vi "GenAppMain.vi"() -> ()   [LabVIEW 2018]
doc: "DESCRIPTION\nGeneral Application \n\nVERSION\nD1:00\nFirst Release To customer\nDD/MM/YYYY\n\nTemplate D2:01\nMade lighter and simpler\n14-04-2020"
uses:
  SubVIs/Controls/SetupModeState.ctl
  <vilib>/event_ctls.llb/eventsource.ctl
  SubVIs/Controls/DisplayQCommand.ctl
  SubVIs/Controls/QueueCommand.ctl
  SubVIs/Controls/DisplayMessage.ctl
  SubVIs/Controls/Transition.ctl
  SubVIs/utilities/Error/ErrorCommand.ctl
  SubVIs/Controls/Tab.ctl
  SubVIs/Controls/StateMessage.ctl
  SubVIs/Error/ErrorMessage.ctl
  SubVIs/utilities/Config/System Config Data Manager Parameter.ctl
  SubVIs/utilities/Config/ConfigCommand.ctl
panel:
  in  "Stop":bool
  in  "Source":T1 items=["LabVIEW UI"=0, "ActiveX"=1, "User Event"=25]
  out "ErrorHandlingLoop":i32
  out "StateMachineLoop":i32
  out "Version":string
  out "Time":string
  out "UILoop":i32
  out "EventLoop":i32
  in  "Main Screen Tabs":enum32{"Main Screen"}(tab)
  out "Tab Control":T2(tab)
  in  "Error Loop":enum16{"Event Loop", "UI Q Loop", "State Loop"}(ring)
  in  "Generate Error":bool
  out "EngMode?":bool
  in  "Enter Password":string
  out "ConfigdB path":path
  in  "Home Button":bool
  in  "ErrorLog":bool
  in  "Clear Alarm":bool
  in  "ErrorLog":i32(listbox)
  out "Error":string
  out "ErrorIndicator":bool
  out "State":T3=enum."Initialising"
  in  "ViewError":bool
  out "Status":string
  in  "Start":bool
  in  "exit":bool
  # "GenAppMain"
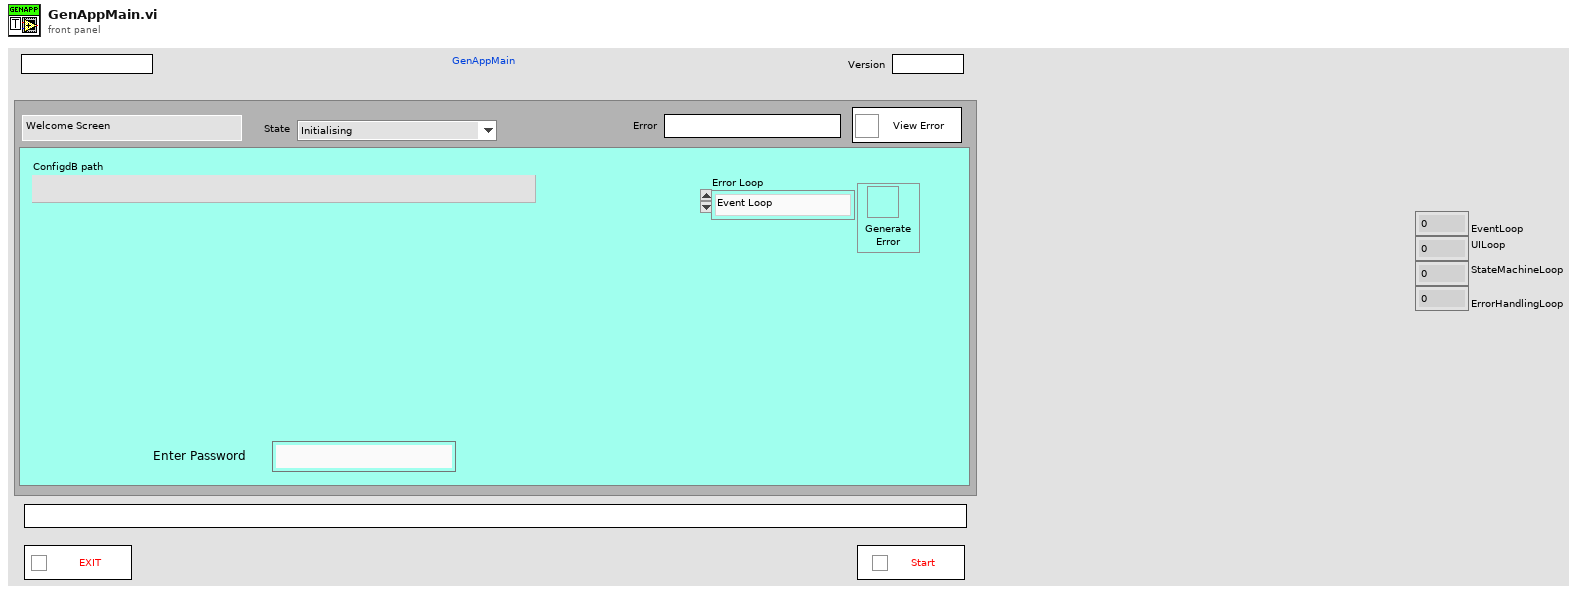
[diagram p1: front panel]
types:
  T1 = typedef "eventsource.ctl" = u32
  T2 = enum32{"Welcome Screen", "Eng Set Up", "Oppo Run Screen", "Eng Run Screen", "Test Report Screen", "Error"}
  T3 = typedef "SetupModeState.ctl" = enum16{"No State - Error", "Initialising", "Idling", "Running", "Erroring", "Exiting"}
  T4 = typedef "DisplayQCommand.ctl" = enum16{"No Command - Error", "Initialise", "Get Q Reference", "Add Item to Bottom", "Add Item to Top", "Flush Q", "Dequeue", "Peek Next Element", "Close"}
  T5 = typedef "QueueCommand.ctl" = enum16{"No Command - Error", "Initialise", "Add to Bottom", "Add To Top", "Get Ref", "Close"}
  T6 = typedef "ErrorCommand.ctl" = enum16{"No Command - Error", "Set to Dev Mode", "Set To Released Mode", "Set Error", "Log Error", "Throw Error", "Log & Throw Error", "Set Error Timed"}
  T7 = enum32{"invalid app kind", "Development System", "Run Time System", "Student Edition", "Embedded LabVIEW", "Evaluation", "Custom"}
  T8 = typedef "DisplayMessage.ctl" = enum16{"No Message - Ignore", "Display Message", "Set Tab", "Set Status", "Add Error Message", "Clear Error History", "Generate Error", "Set Idling Display", "Set Running Display", "Stop"}
  T9 = typedef "ErrorMessage.ctl" = enum16{"No Message - Ignore", "Display Message", "Stop"}
  T10 = typedef "StateMessage.ctl" = cluster{"Transition":T11, "variant":variant}
  T11 = typedef "Transition.ctl" = enum16{"No Transition - Error", "Initialise", "Login", "Authenticate", "Log on Fail", "Login Success", "Logout", "Generate Error", "Start", "Stop", "Exit"}
  T12 = typedef "ConfigCommand.ctl" = enum16{"No Command - Error", "Initialise Config SQLite", "Save Config", "Get Key", "Set Key", "Update Key", "Get Latest Config Data", "Get Config Data for Version", "Get Default Config Data"}
  T13 = typedef "System Config Data Manager Parameter.ctl" = enum16{"Eng Password", "DSN Connection", "User Password", "RunStatus", "InitialDataPath", "helpFilePath", "ErrorFilepath", "DatalogPath", "Hello"}
  T14 = typedef "Tab.ctl" = enum32{"Welcome Screen", "Eng Set Up", "Oppo Run Screen", "Eng Run Screen", "Test Report Screen", "Error"}
  T15 = typedef "lveventtype.ctl" = enum32{"Null", "Timeout", "Annotation Menu Selection", "Annotation Menu Selection?", "App Instance Close", "App Instance Close?", "Autoscale Range Change", "Bookmark Info Change", "Cell Edit", "Cell Edit?", "Cursor Grab", "Cursor Grab?", "Cursor Menu Selection", "Cursor Menu Selection?", "Cursor Move", "Cursor Release", "Data Change", "Direction Change", "Display State Change", "Drag Ended", "Drag Enter", "Drag Leave", "Drag Over", "Drag Source Update", "Drag Starting", "Drag Starting?", "Drop", "Exec State Change", "Key Down", "Key Down?", "Key Repeat", "Key Repeat?", "Key Up", "Listbox Double Click", "Menu Activation?", "Menu Selection (App)", "Menu Selection? (App)", "Menu Selection (User)", "Mouse Down", "Mouse Down?", "Mouse Enter", "Mouse Leave", "Mouse Move", "Mouse Up", "Mouse Wheel", "NI Security User Change (App)", "Pane Size", "Panel Close", "Panel Close?", "Panel Resize", "Plot Attribute Change", "Scale Range Change", "Shortcut Menu Activation?", "Shortcut Menu Selection (App)", "Shortcut Menu Selection? (App)", "Shortcut Menu Selection (User)", "Tree Double Click", "Tree Drag", "Tree Drag?", "Tree Drop", "Tree Drop?", "Tree Item Close", "Tree Item Close?", "Tree Item Open", "Tree Item Open?", "User Event", "Value Change"}
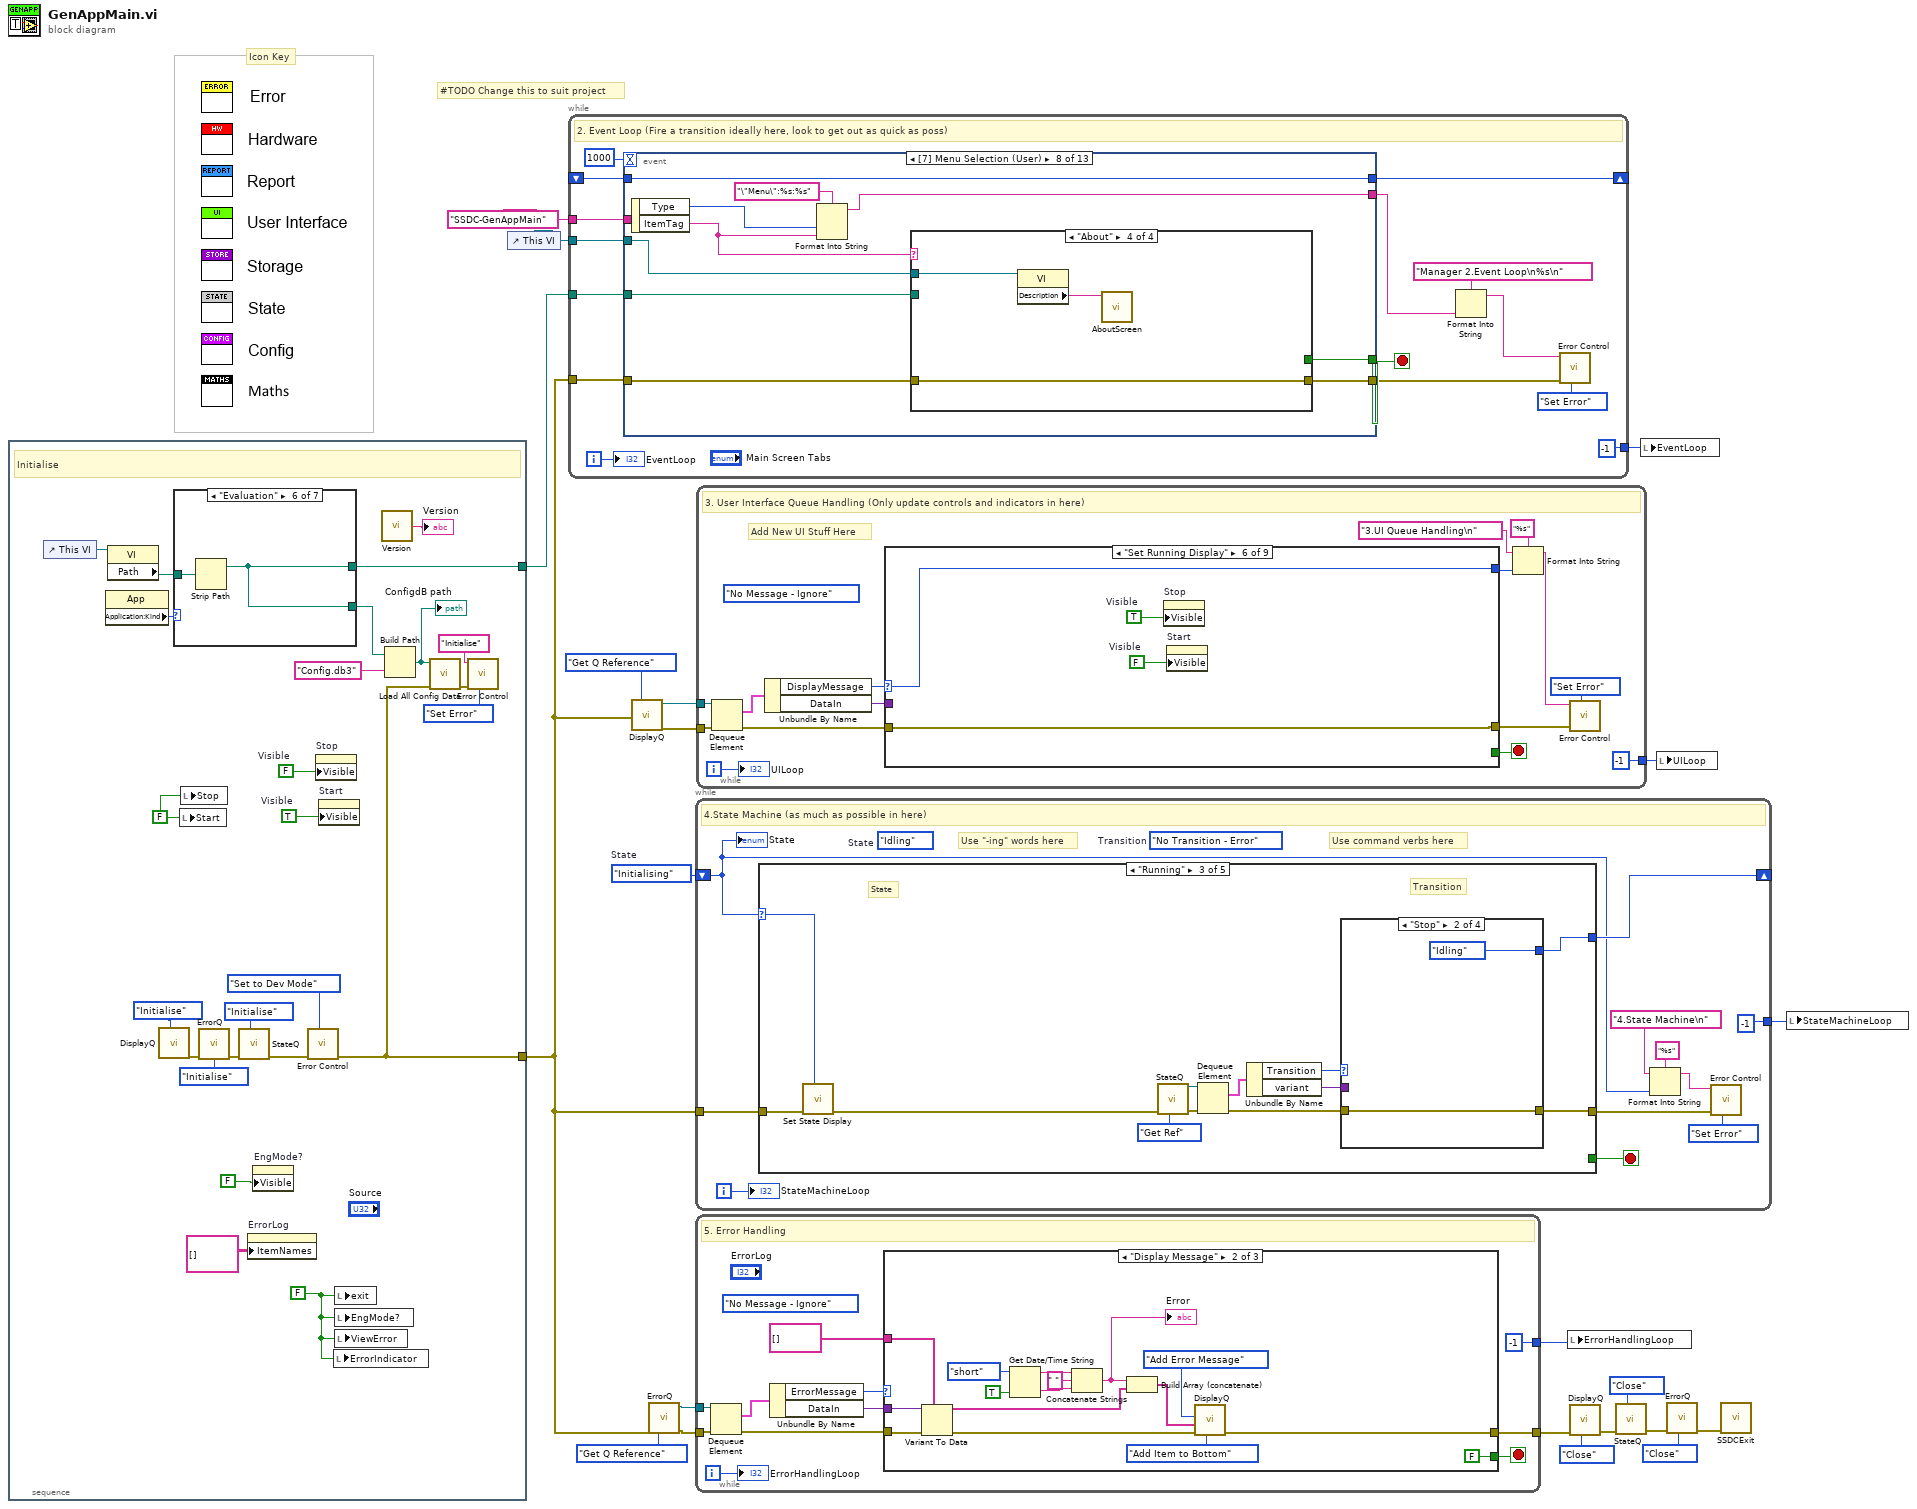
[diagram p0: block diagram]
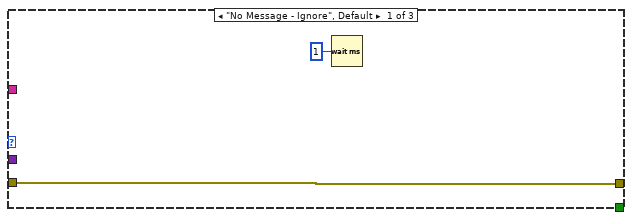
[diagram p2: hidden frame]
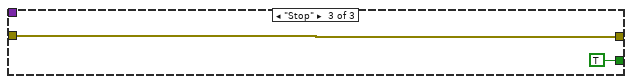
[diagram p3: hidden frame]
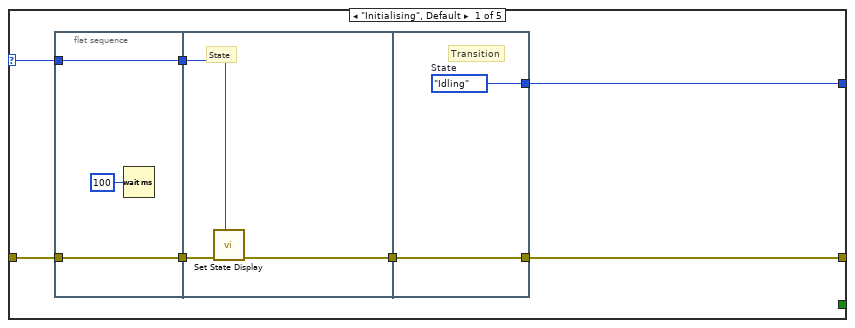
[diagram p4: hidden frame]
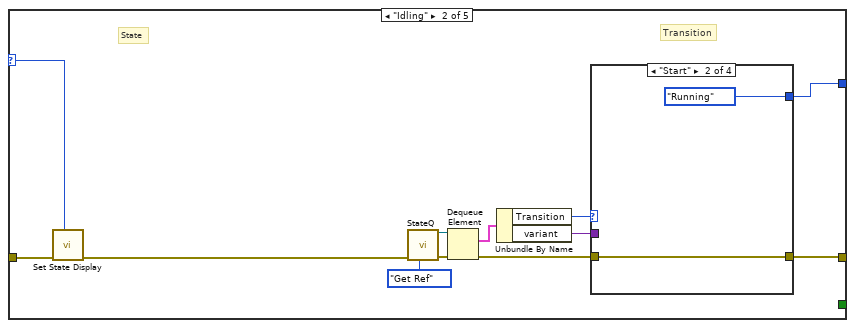
[diagram p5: hidden frame]
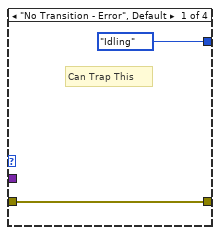
[diagram p6: hidden frame]
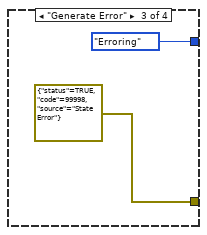
[diagram p7: hidden frame]
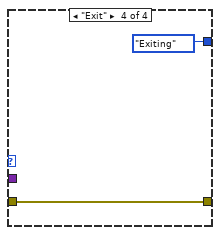
[diagram p8: hidden frame]
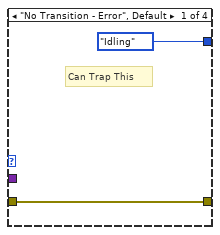
[diagram p9: hidden frame]
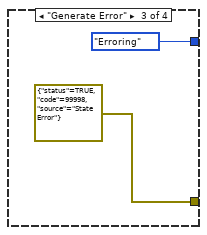
[diagram p10: hidden frame]
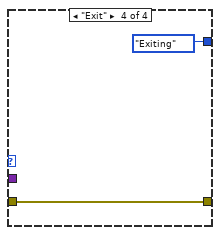
[diagram p11: hidden frame]
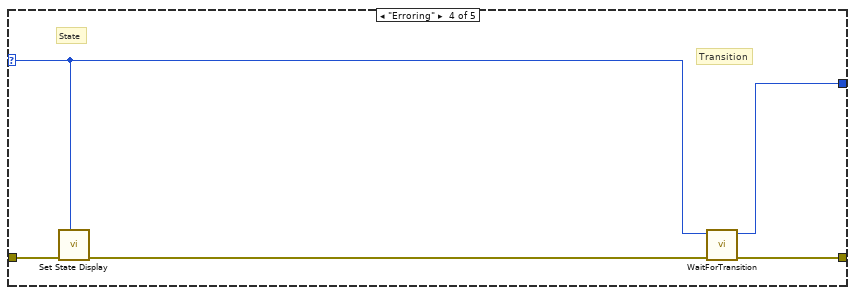
[diagram p12: hidden frame]
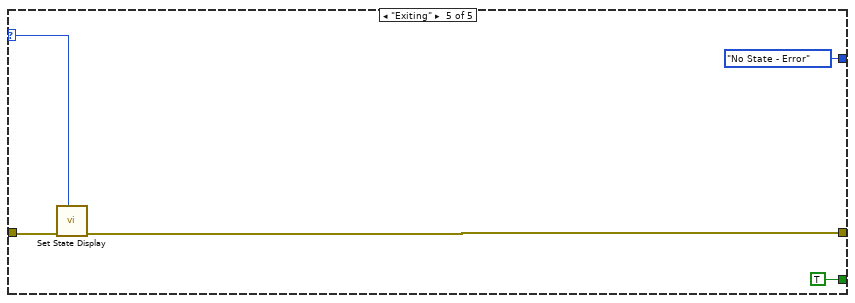
[diagram p13: hidden frame]
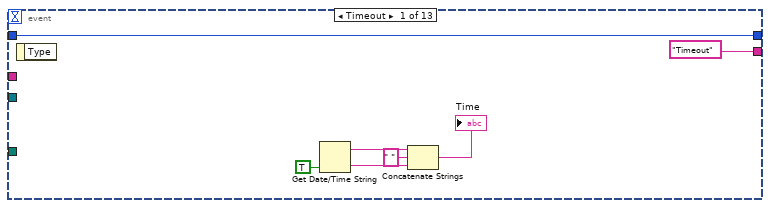
[diagram p14: hidden frame]
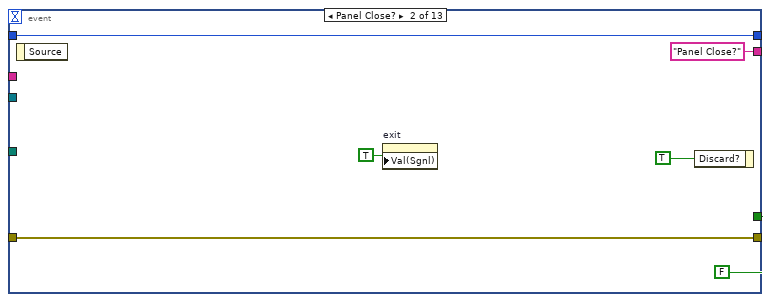
[diagram p15: hidden frame]
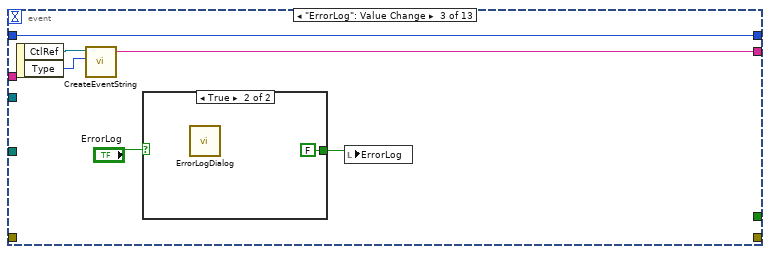
[diagram p16: hidden frame]
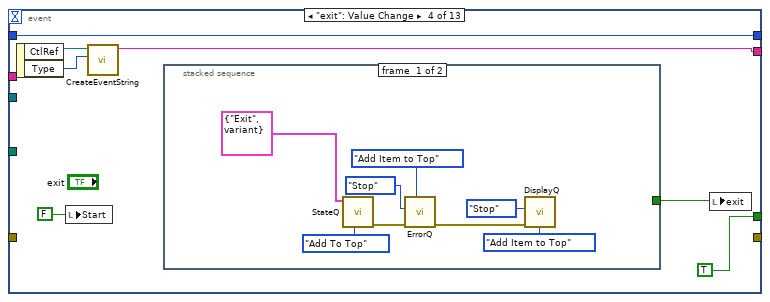
[diagram p18: hidden frame]
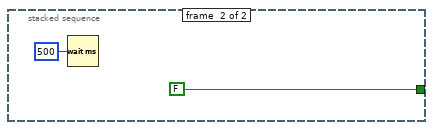
[diagram p19: hidden frame]
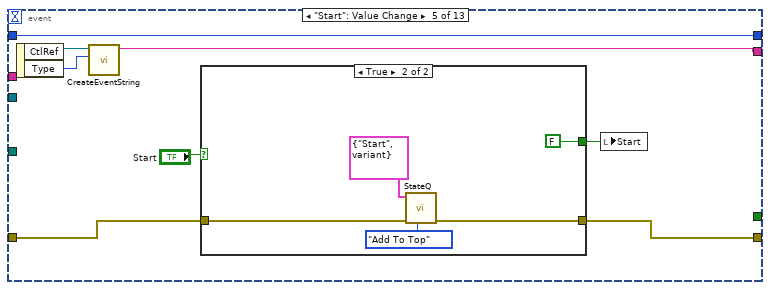
[diagram p20: hidden frame]
diagram:
  w22 = SetupModeState."Initialising"  # State
  # "#TODO Change this to suit project"
  # "Icon Key"
  n1 = stacked-sequence "1. Initialisation" {
    tunnel: [w26] -> w8
    tunnel: [w31] -> w16
    frame #0 {
      w24 = FALSE  # Visible
      w23 = TRUE  # Visible
      w29 = FALSE ("Stopped")
      w25 = FALSE ("Start")
      # "Initialise"
      n2 = control-ref of="This VI"() -> (w42:refnum<vi>)
      n3 = property class="App"() -> ("Application:Kind"=w41:T7)  [unwired: 2 in, 2 out]
      n4 = property class="VI"(reference=w42) -> ("Path"=w43:path)  [unwired: 1 in, 2 out]
      n5 = call "DisplayQ.vi"("command"=DisplayQCommand."Initialise") -> ("error out"=w36:errorcluster)  [unwired: 4 in, 3 out]
      n6 = case shown="\"Evaluation\"" w41 {
        tunnel: w43 -> [w48 w50 w54 w57 w59 w61 w63]
        tunnel: [w48 w49 w53 w56 w58 w60 w62] -> w32
        tunnel: [w48 w49 w51 w56 w58 w60 w62] -> w31
        frame "invalid app kind", Default {
        }
        frame "Development System" {
          n7 = Strip Path(path=w50) -> (stripped path=w49:path)  [unwired: 1 out]
        }
        frame "Run Time System" {
          n8 = Strip Path(path=w54) -> (stripped path=w55:path)  [unwired: 1 out]
          n9 = Strip Path(path=w55) -> (stripped path=w51:path)  [unwired: 1 out]
          n10 = Build Path(base path=w51, name or relative path="data") -> (appended path=w53:path)
        }
        frame "Student Edition" {
          n11 = Strip Path(path=w57) -> (stripped path=w56:path)  [unwired: 1 out]
        }
        frame "Embedded LabVIEW" {
          n12 = Strip Path(path=w59) -> (stripped path=w58:path)  [unwired: 1 out]
        }
        frame "Evaluation" {
          n13 = Strip Path(path=w61) -> (stripped path=w60:path)  [unwired: 1 out]
        }
        frame "Custom" {
          n14 = Strip Path(path=w63) -> (stripped path=w62:path)  [unwired: 1 out]
        }
      }
      n15 = local write "Start"(w25) -> ()
      n16 = local write "Stop"(w25) -> ()
      n17 = call "ErrorQ.vi"("command"=DisplayQCommand."Initialise", "error in (no error)"=w36) -> ("error out"=w37:errorcluster)  [unwired: 3 in, 3 out]
      n18 = call "StateQ.vi"("QueueCommand"=QueueCommand."Initialise", "error in (no error)"=w37) -> ("error out"=w27:errorcluster)  [unwired: 5 in, 1 out]
      n19 = property on="ErrorLog" class="MCListbox (strict)"("ItemNames"=string[][] [] ("Item Names")) -> ()  [unwired: 2 in, 2 out]
      n20 = property on="EngMode?" class="Bool (strict)"("Visible"=FALSE) -> ()  [unwired: 2 in, 2 out]
      n21 = call "Error Control.vi"("Command"=ErrorCommand."Set to Dev Mode", "error in (no error)"=w27) -> ("error out"=w26:errorcluster)  [unwired: 6 in]
      n22 = property on="Stop" class="Bool (strict)"("Visible"=w24) -> ()  [unwired: 2 in, 2 out]
      n23 = property on="Start" class="Bool (strict)"("Visible"=w23) -> ()  [unwired: 2 in, 2 out]
      n24 = local write "ErrorIndicator"(w29) -> ()
      n25 = local write "exit"(w29) -> ()
      n26 = local write "EngMode?"(w29) -> ()
      n27 = local write "ViewError"(w29) -> ()
      n28 = call "Version.vi"() -> ("Version"=→"Version":string)  [unwired: 5 in]
      n29 = Build Path(base path=w32, name or relative path="Config.db3") -> (appended path=w44:path)
      "ConfigdB path" <- w44
      n30 = call "Load All Config Data.vi"("error in (no error)"=w26, "path"=w44) -> ("error out"=w34:errorcluster)  [unwired: 5 in]
      n31 = call "Error Control.vi"("Command"=ErrorCommand."Set Error", "error in (no error)"=w34, "Source"="Initialise") -> ()  [unwired: 5 in, 1 out]
    }
  }
  n32 = control-ref of="This VI"() -> (w21:refnum<vi>)
  n33 = while "2. Event Loop" {
    tunnel: w8 -> [w75]
    shift-right: [w72] -> _
    shift-left: _ -> [w71]
    tunnel: w21 -> [w70]
    tunnel: [-1 ("ErrorHandlingLoop")] -> w17
    tunnel: w16 -> [w68]
    tunnel: "SSDC-GenAppMain" ("name or relative path") -> [w67]
    i -> [w78]
    stop <- w77 stop-if-true
    # "2. Event Loop (Fire a transition ideally here, look to get out as quick as poss)"
    n34 = event shown="[7] Menu Selection (User)" {
      selector: _ -> [_ _ _ _ _ _ _ _ _ _ _ _ _]
      dyn-events: _ -> [_ _ _ _ _ _ _ _ _ _ _ _ _]
      timeout: 1000 -> [_ _ _ _ _ _ _ _ _ _ _ _ _]
      tunnel: [_ FALSE ("STOP?") _ TRUE ("STOP?") _ _ _ w162 _ _ _ _ _] -> w77
      tunnel: w75 -> [_ w88 _ _ w120 w135 _ w159 w179 w197 w210 w233 _]
      tunnel: [_ w88 _ _ w119 w134 _ w158 w178 w196 w209 w232 _] -> w73
      tunnel: ["Timeout" "Panel Close?" ("Event") w92 w99 w116 w130 w144 w153 w171 w190 w203 w226 w245] -> w64
      tunnel: [w80 w87 w97 w102 w123 w137 w147 w161 w174 w195 w206 w234 w249] -> w72
      tunnel: w71 -> [w80 w87 w97 w102 w123 w137 w147 w161 _ w195 w206 w234 w249]
      tunnel: w70 -> [_ _ _ _ _ _ _ w160 _ _ _ _ w248]
      tunnel: w68 -> [_ _ _ _ _ _ _ w157 _ _ _ _ _]
      tunnel: w67 -> [_ _ _ _ _ _ _ _ _ _ _ _ _]
      event Timeout {
        n35 = event-data() -> ()  [unwired: 1 in, 1 out]
        n36 = Get Date/Time String(want seconds? (F)=TRUE) -> (date string=w84:string, time string=w83:string)  [unwired: 2 in]
        n37 = Concatenate Strings(w84, " " ("string"), w83) -> (→"Time":string)
      }
      event Panel Close? {
        n38 = event-data() -> ()  [unwired: 1 in, 1 out]
        n39 = property on="exit" class="Bool (strict)"("Val(Sgnl)"=TRUE ("Value (Signaling)")) -> ()  [unwired: 2 in, 2 out]
        n40 = event-data("Discard?"=TRUE) -> ()  [unwired: 1 in, 1 out]
      }
      event "ErrorLog": Value Change {
        n41 = event-data() -> ("CtlRef"=w94:refnum<vi>, "Type"=w93:T15)  [unwired: 1 in]
        n42 = call "CreateEventString.vi"("Type in"=w93, "Ctl Refnum"=w94) -> ("Event"=w92:string)  [unwired: 9 in]
        n43 = case shown="True" "ErrorLog" {
          tunnel: [_ FALSE] -> w95
          frame False {
          }
          frame True {
            n44 = call "ErrorLogDialog.vi"() -> ()  [unwired: 11 in, 1 out]
          }
        }
        n45 = local write "ErrorLog"(w95) -> ()
      }
      event "exit": Value Change {
        n46 = event-data() -> ("CtlRef"=w101:refnum<vi>, "Type"=w100:T15)  [unwired: 1 in]
        n47 = local write "Start"(FALSE ("Start")) -> ()
        n48 = call "CreateEventString.vi"("Type in"=w100, "Ctl Refnum"=w101) -> ("Event"=w99:string)  [unwired: 9 in]
        n49 = stacked-sequence {
          tunnel: [_ FALSE] -> w103
          frame #0 {
            n50 = call "StateQ.vi"("QueueCommand"=QueueCommand."Add To Top", "output cluster"=T10 {"Transition"=enum."Exit", "variant"=variant}) -> ("error out"=w110:errorcluster)  [unwired: 5 in, 1 out]
            n51 = call "ErrorQ.vi"("command"=DisplayQCommand."Add Item to Top", "error in (no error)"=w110, "ErrorMessage"=ErrorMessage."Stop") -> ("error out"=w107:errorcluster)  [unwired: 2 in, 3 out]
            n52 = call "DisplayQ.vi"("command"=DisplayQCommand."Add Item to Top", "error in (no error)"=w107, "DisplayMessage"=DisplayMessage."Stop") -> ()  [unwired: 2 in, 4 out]
          }
          frame #1 {
            n53 = Wait (ms)(milliseconds to wait=u32 500) -> ()  [unwired: 1 out]
          }
        }
        n54 = local write "exit"(w103) -> ()
      }
      event "Start": Value Change {
        n55 = event-data() -> ("CtlRef"=w118:refnum<vi>, "Type"=w117:T15)  [unwired: 1 in]
        n56 = call "CreateEventString.vi"("Type in"=w117, "Ctl Refnum"=w118) -> ("Event"=w116:string)  [unwired: 9 in]
        n57 = case shown="True" "Start" {
          tunnel: [_ FALSE ("Start")] -> w121
          tunnel: w120 -> [w124 w126]
          tunnel: [w124 w125] -> w119
          frame False {
          }
          frame True {
            n58 = call "StateQ.vi"("QueueCommand"=QueueCommand."Add To Top", "error in (no error)"=w126, "output cluster"=T10 {"Transition"=enum."Start", "variant"=variant}) -> ("error out"=w125:errorcluster)  [unwired: 4 in, 1 out]
          }
        }
        n59 = local write "Start"(w121) -> ()
      }
      event "Stop": Value Change {
        n60 = event-data() -> ("CtlRef"=w132:refnum<vi>, "Type"=w131:T15)  [unwired: 1 in]
        n61 = call "CreateEventString.vi"("Type in"=w131, "Ctl Refnum"=w132) -> ("Event"=w130:string)  [unwired: 9 in]
        n62 = case shown="True" "Stop" {
          tunnel: [_ FALSE ("Start")] -> w136
          tunnel: w135 -> [w138 w140]
          tunnel: [w138 w139] -> w134
          frame False {
          }
          frame True {
            n63 = call "StateQ.vi"("QueueCommand"=QueueCommand."Add To Top", "error in (no error)"=w140, "output cluster"=T10 {"Transition"=enum."Stop", "variant"=variant}) -> ("error out"=w139:errorcluster)  [unwired: 4 in, 1 out]
          }
        }
        n64 = local write "Stop"(w136) -> ()
      }
      event "Enter Password": Value Change {
        n65 = event-data() -> ("CtlRef"=w146:refnum<vi>, "Type"=w145:T15)  [unwired: 1 in]
        n66 = call "CreateEventString.vi"("Type in"=w145, "Ctl Refnum"=w146) -> ("Event"=w144:string)  [unwired: 9 in]
        n67 = call "SQLiteConfig.vi"("ConfigCommand"=ConfigCommand."Get Key", "Parameter"=System_Config_Data_Manager_Parameter."Eng Password") -> ("KeyData"=w148:string)  [unwired: 3 in, 3 out]
        n68 = Equal?(x=w148, y="Enter Password") -> (x = y?=w152:bool)
        "EngMode?" <- w152
        n69 = property on="EngMode?" class="Bool (strict)"("Visible"=w152) -> ()  [unwired: 2 in, 2 out]
      }
      event Menu Selection (User) {
        n70 = event-data() -> ("Type"=w155:T15, "ItemTag"=w154:string)  [unwired: 1 in]
        n71 = Format Into String(format string="\"Menu\":%s:%s", w155, w154) -> (resulting string=w153:string)  [unwired: 2 in, 1 out]
        n72 = case shown="\"About\"" w154 {
          tunnel: [_ FALSE _ _] -> w162
          tunnel: w160 -> [_ _ _ w170]
          tunnel: w159 -> [w163 w164 w167 w168]
          tunnel: [w163 w164 w167 w168] -> w158
          tunnel: w157 -> [_ _ _ _]
          frame "False", Default {
          }
          frame "Exit" {
            n73 = property on="exit" class="Bool (strict)"("Val(Sgnl)"=TRUE ("Value (Signaling)")) -> ()  [unwired: 2 in, 2 out]
          }
          frame "Configuration" {
            n74 = call "ConfigSQLiteSettingDialog.vi"() -> ()  [unwired: 1 in]
          }
          frame "About" {
            n75 = property class="VI"(reference=w170) -> ("Description"=w169:string)  [unwired: 1 in, 2 out]
            n76 = call "AboutScreen.vi"("Version Info. In"=w169) -> ()  [unwired: 11 in]
          }
        }
      }
      event "ViewError": Value Change {
        n77 = event-data() -> ("CtlRef"=w172:refnum<vi>, "Type"=w173:T15)  [unwired: 1 in]
        n78 = local read "Tab Control"() -> (w175:T2)
        n79 = call "CreateEventString.vi"("Type in"=w173, "Ctl Refnum"=w172) -> ("Event"=w171:string)  [unwired: 9 in]
        n80 = case shown="True" "ViewError" {
          tunnel: w179 -> [w182 w186]
          tunnel: [w182 w185] -> w178
          tunnel: [FALSE FALSE] -> w176
          tunnel: w175 -> [w180 w183]
          tunnel: [w180 w183] -> w174
          frame False {
          }
          frame True {
            n81 = call "DisplayQ.vi"("command"=DisplayQCommand."Add Item to Bottom", "error in (no error)"=w186, "DataIn"=Tab."Error" ("Tab Control"), "DisplayMessage"=DisplayMessage."Set Tab") -> ("error out"=w185:errorcluster)  [unwired: 1 in, 3 out]
          }
        }
        n82 = local write "ViewError"(w176) -> ()
      }
      event "Clear Alarm": Value Change {
        n83 = event-data() -> ("CtlRef"=w191:refnum<vi>, "Type"=w192:T15)  [unwired: 1 in]
        n84 = call "CreateEventString.vi"("Type in"=w192, "Ctl Refnum"=w191) -> ("Event"=w190:string)  [unwired: 9 in]
        n85 = case shown="True" "Clear Alarm" {
          tunnel: w197 -> [w199 w201]
          tunnel: [w199 w201] -> w196
          tunnel: [FALSE FALSE] -> w193
          frame False {
          }
          frame True {
            n86 = local write "ErrorIndicator"(FALSE ("ErrorIndicator")) -> ()
          }
        }
        n87 = local write "Clear Alarm"(w193) -> ()
      }
      event "Home Button": Value Change {
        n88 = event-data() -> ("CtlRef"=w205:refnum<vi>, "Type"=w204:T15)  [unwired: 1 in]
        n89 = call "CreateEventString.vi"("Type in"=w204, "Ctl Refnum"=w205) -> ("Event"=w203:string)  [unwired: 9 in]
        n90 = case shown="True" "Home Button" {
          tunnel: w210 -> [w212 w217]
          tunnel: [w212 w216] -> w209
          tunnel: [FALSE FALSE] -> w208
          tunnel: w206 -> [_ w214]
          frame False {
          }
          frame True {
            n91 = case shown="\"Error\"" w214 {
              tunnel: [Tab."Welcome Screen" ("Tab Control") Tab."Oppo Run Screen" ("Tab Control") Tab."Eng Run Screen" ("Tab Control") Tab."Test Report Screen" ("Tab Control") Tab."Error" ("Tab Control") Tab."Eng Run Screen" ("Tab Control")] -> w213
              frame "Welcome Screen" {
              }
              frame "Oppo Run Screen" {
              }
              frame "Eng Run Screen" {
              }
              frame "Test Report Screen" {
              }
              frame "Error" {
              }
              frame "Eng Set Up" {
              }
            }
            n92 = call "DisplayQ.vi"("command"=DisplayQCommand."Add Item to Bottom", "error in (no error)"=w217, "DataIn"=w213, "DisplayMessage"=DisplayMessage."Set Tab") -> ("error out"=w216:errorcluster)  [unwired: 1 in, 3 out]
          }
        }
        n93 = local write "Home Button"(w208) -> ()
      }
      event "Generate Error": Value Change {
        n94 = event-data() -> ("CtlRef"=w228:refnum<vi>, "Type"=w227:T15)  [unwired: 1 in]
        n95 = call "CreateEventString.vi"("Type in"=w227, "Ctl Refnum"=w228) -> ("Event"=w226:string)  [unwired: 9 in]
        n96 = case shown="\"UI Q Loop\"" "Error Loop" {
          tunnel: w233 -> [_ w237 w242]
          tunnel: [errorcluster {"status"=TRUE, "code"=99999, "source"="Random Event Error"} ("error out") w236 w243] -> w232
          tunnel: "Generate Error" -> [_ _ _]
          tunnel: [_ _ FALSE] -> w229
          frame "Event Loop", Default {
          }
          frame "UI Q Loop" {
            n97 = call "DisplayQ.vi"("command"=DisplayQCommand."Add Item to Bottom", "error in (no error)"=w237, "DisplayMessage"=DisplayMessage."Generate Error") -> ("error out"=w236:errorcluster)  [unwired: 2 in, 3 out]
          }
          frame "State Loop" {
            n98 = call "StateQ.vi"("QueueCommand"=QueueCommand."Add to Bottom", "error in (no error)"=w242, "output cluster"=T10 {"Transition"=enum."Generate Error", "variant"=variant}) -> ("error out"=w243:errorcluster)  [unwired: 4 in, 1 out]
          }
        }
        n99 = local write "Generate Error"(w229) -> ()
      }
      event "Version": Mouse Down {
        n100 = event-data() -> ("CtlRef"=w247:refnum<vi>, "Type"=w246:T15)  [unwired: 1 in]
        n101 = call "CreateEventString.vi"("Type in"=w246, "Ctl Refnum"=w247) -> ("Event"=w245:string)  [unwired: 9 in]
        n102 = property class="VI"(reference=w248) -> ("Description"=w250:string)  [unwired: 1 in, 2 out]
        n103 = call "VIDescription.vi"("VersionData In"=w250) -> ()  [unwired: 10 in, 1 out]
      }
    }
    n104 = Format Into String(format string="Manager 2.Event Loop\n%s\n", w64) -> (resulting string=w65:string)  [unwired: 2 in, 1 out]
    n105 = call "Error Control.vi"("Command"=ErrorCommand."Set Error", "error in (no error)"=w73, "Source"=w65) -> ()  [unwired: 5 in, 1 out]
    "EventLoop" <- w78
  }
  n106 = call "DisplayQ.vi"("command"=DisplayQCommand."Get Q Reference", "error in (no error)"=w8) -> ("error out"=w10:errorcluster, "queue out"=w11:refnum<queue>)  [unwired: 3 in, 2 out]
  n107 = call "ErrorQ.vi"("command"=DisplayQCommand."Get Q Reference", "error in (no error)"=w8) -> ("error out"=w13:errorcluster, "queue out"=w14:refnum<queue>)  [unwired: 3 in, 2 out]
  n108 = while {
    shift-right: [w259] -> _
    shift-left: w22 -> [w255]
    tunnel: w8 -> [w260]
    tunnel: [-1 ("ErrorHandlingLoop")] -> w19
    i -> [w258]
    stop <- w261 stop-if-true
    (unwired) SetupModeState."Idling"  # State
    (unwired) Transition."No Transition - Error"  # Transition
    # "Use command verbs here"
    # "Use \"-ing\" words here"
    # "4.State Machine (as much as possible in here)"
    n109 = case shown="\"Running\"" w255 {
      selector: w255 -> [w267 w287 w307 w317 w323]
      tunnel: [_ _ _ _ TRUE] -> w261
      tunnel: w260 -> [w268 w288 w308 w321 w324]
      tunnel: [w266 w278 w298 w320 SetupModeState."No State - Error" ("State 2")] -> w259
      tunnel: [w265 w279 w299 w319 w322] -> w256
      frame "Initialising", Default {
        n110 = flat-sequence {
          tunnel: w267 -> [w270]
          tunnel: w268 -> [w271]
          tunnel: [w271] -> w263
          tunnel: [w270] -> w262
          tunnel: [w272] -> w264
          tunnel: w263 -> [w274]
          tunnel: w262 -> [w273]
          tunnel: [w276] -> w266
          tunnel: [w275] -> w265
          tunnel: w264 -> [w275]
          frame #0 {
            n111 = Wait (ms)(milliseconds to wait=u32 100) -> ()  [unwired: 1 out]
          }
          frame #1 {
            # "State"
            n112 = call "Set State Display.vi"("State"=w273, "error in (no error)"=w274) -> ("error out"=w272:errorcluster)  [unwired: 6 in]
          }
          frame #2 {
            w276 = SetupModeState."Idling"  # State
            # "Transition"
          }
        }
      }
      frame "Idling" {
        # "Transition"
        # "State"
        n113 = call "Set State Display.vi"("State"=w287, "error in (no error)"=w288) -> ("error out"=w282:errorcluster)  [unwired: 6 in]
        n114 = call "StateQ.vi"("QueueCommand"=QueueCommand."Get Ref", "error in (no error)"=w282) -> ("error out"=w284:errorcluster, "queue out"=w283:refnum<queue>)  [unwired: 5 in]
        n115 = Dequeue Element(queue=w283, error in (no error)=w284) -> (element=w286:T10, error out=w281:errorcluster)  [unwired: 1 in, 2 out]
        n116 = Unbundle By Name(w286) -> ("Transition"=w280:T11, "variant"=w277:variant)
        n117 = case shown="\"Start\"" w280 {
          tunnel: [SetupModeState."Idling" ("State 2") SetupModeState."Running" ("State 2") SetupModeState."Erroring" ("State 2") SetupModeState."Exiting" ("State 2")] -> w278
          tunnel: w281 -> [w289 w291 _ w295]
          tunnel: [w289 w291 errorcluster {"status"=TRUE, "code"=99998, "source"="State Error"} ("error out") w295] -> w279
          tunnel: w277 -> [_ _ _ _]
          frame "No Transition - Error", Default {
            # "Can Trap This"
          }
          frame "Start" {
          }
          frame "Generate Error" {
          }
          frame "Exit" {
          }
        }
      }
      frame "Running" {
        # "Transition"
        # "State"
        n118 = call "Set State Display.vi"("State"=w307, "error in (no error)"=w308) -> ("error out"=w302:errorcluster)  [unwired: 6 in]
        n119 = call "StateQ.vi"("QueueCommand"=QueueCommand."Get Ref", "error in (no error)"=w302) -> ("error out"=w304:errorcluster, "queue out"=w303:refnum<queue>)  [unwired: 5 in]
        n120 = Dequeue Element(queue=w303, error in (no error)=w304) -> (element=w306:T10, error out=w301:errorcluster)  [unwired: 1 in, 2 out]
        n121 = Unbundle By Name(w306) -> ("Transition"=w300:T11, "variant"=w297:variant)
        n122 = case shown="\"Stop\"" w300 {
          tunnel: [SetupModeState."Idling" ("State 2") SetupModeState."Idling" ("State 2") SetupModeState."Erroring" ("State 2") SetupModeState."Exiting" ("State 2")] -> w298
          tunnel: w301 -> [w309 w311 _ w315]
          tunnel: [w309 w311 errorcluster {"status"=TRUE, "code"=99998, "source"="State Error"} ("error out") w315] -> w299
          tunnel: w297 -> [_ _ _ _]
          frame "No Transition - Error", Default {
            # "Can Trap This"
          }
          frame "Stop" {
          }
          frame "Generate Error" {
          }
          frame "Exit" {
          }
        }
      }
      frame "Erroring" {
        # "Transition"
        # "State"
        n123 = call "Set State Display.vi"("State"=w317, "error in (no error)"=w321) -> ("error out"=w318:errorcluster)  [unwired: 6 in]
        n124 = call "WaitForTransition.vi"("error in (no error)"=w318, "State"=w317) -> ("error out"=w319:errorcluster, "StateOut"=w320:T3)  [unwired: 4 in]
      }
      frame "Exiting" {
        n125 = call "Set State Display.vi"("State"=w323, "error in (no error)"=w324) -> ("error out"=w322:errorcluster)  [unwired: 6 in]
      }
    }
    n126 = Format Into String(format string="%s", initial string="4.State Machine\n", w255) -> (resulting string=w254:string)  [unwired: 1 in, 1 out]
    n127 = call "Error Control.vi"("Command"=ErrorCommand."Set Error", "error in (no error)"=w256, "Source"=w254) -> ()  [unwired: 5 in, 1 out]
    "StateMachineLoop" <- w258
    "State" <- w255
  }
  n128 = while {
    tunnel: w13 -> [w337]
    tunnel: w14 -> [w336]
    tunnel: [w328] -> w1
    tunnel: [-1 ("ErrorHandlingLoop")] -> w20
    i -> [w330]
    stop <- w331 stop-if-true
    (unwired) DisplayMessage."No Message - Ignore" ("DisplayMessage")
    # "5. Error Handling"
    n129 = Dequeue Element(queue=w336, error in (no error)=w337) -> (element=w335:cluster{"ErrorMessage":T9, "DataIn":variant}, error out=w332:errorcluster)  [unwired: 1 in, 2 out]
    n130 = Unbundle By Name(w335) -> ("ErrorMessage"=w333:T9, "DataIn"=w334:variant)
    n131 = case shown="\"Display Message\"" w333 {
      tunnel: w334 -> [_ w354 _]
      tunnel: w332 -> [w338 w353 w357]
      tunnel: [w338 w344 w357] -> w328
      tunnel: [_ FALSE ("STOP?") TRUE ("STOP?")] -> w331
      tunnel: string[] [] -> [_ w352 _]
      frame "No Message - Ignore", Default {
        n132 = Wait (ms)(milliseconds to wait=u32 1) -> ()  [unwired: 1 out]
      }
      frame "Display Message" {
        n133 = Variant To Data(error in=w353, type=w352, Variant=w354) -> (data=w346:string[], error out=w345:errorcluster)
        n134 = Get Date/Time String(date format (0)=enum16{"short", "long", "abbreviated"}."short", want seconds? (F)=TRUE) -> (date string=w349:string, time string=w348:string)  [unwired: 1 in]
        n135 = Concatenate Strings(w349, " " ("string"), w348) -> (w340:string)
        "Error" <- w340
        n136 = Build Array (concatenate)(w340, w346) -> (w341:string[])
        n137 = call "DisplayQ.vi"("command"=DisplayQCommand."Add Item to Bottom", "error in (no error)"=w345, "DataIn"=w341, "DisplayMessage"=DisplayMessage."Add Error Message") -> ("error out"=w344:errorcluster)  [unwired: 1 in, 3 out]
      }
      frame "Stop" {
      }
    }
    "ErrorHandlingLoop" <- w330
  }
  n138 = while "3. User Interface Queue Handling" {
    tunnel: w10 -> [w372]
    tunnel: w11 -> [w371]
    tunnel: [-1 ("ErrorHandlingLoop")] -> w18
    i -> [w363]
    stop <- w364 stop-if-true
    (unwired) DisplayMessage."No Message - Ignore" ("DisplayMessage")
    # "Add New UI Stuff Here"
    # "3. User Interface Queue Handling (Only update controls and indicators in here)"
    n139 = Dequeue Element(queue=w371, error in (no error)=w372) -> (element=w370:cluster{"DisplayMessage":T8, "DataIn":variant}, error out=w367:errorcluster)  [unwired: 1 in, 2 out]
    n140 = Unbundle By Name(w370) -> ("DisplayMessage"=w368:T8, "DataIn"=w369:variant)
    n141 = case shown="\"Set Running Display\"" w368 {
      selector: w368 -> [w373 w376 w379 w394 w401 w405 w409 w411 w413]
      tunnel: w369 -> [_ _ w388 w397 _ _ _ _ w417]
      tunnel: w367 -> [w374 w378 w381 w396 w400 w404 w408 _ w415]
      tunnel: [w374 w378 w380 w395 w400 w404 w408 errorcluster {"status"=TRUE, "code"=99997, "source"="UI Error"} ("error out") w414] -> w366
      tunnel: [_ TRUE ("STOP?") _ _ _ _ _ _ _] -> w364
      tunnel: [w373 w376 w379 w394 w401 w405 w409 w411 w413] -> w362
      frame "No Message - Ignore", Default {
        n142 = Wait (ms)(milliseconds to wait=u32 1) -> ()  [unwired: 1 out]
      }
      frame "Stop" {
      }
      frame "Display Message" {
        n143 = Variant To Data(error in=w381, type="" ("data"), Variant=w388) -> (data=w384:string, error out=w380:errorcluster)
        n144 = local read "State"() -> (w386:T3)
        n145 = Format Into String(w386) -> (resulting string=w385:string)  [unwired: 3 in, 1 out]
        n146 = Concatenate Strings(w385, " - " ("string"), w384) -> (→"Status":string)
      }
      frame "Add Error Message" {
        n147 = property on="ErrorLog" class="MCListbox (strict)"() -> ("ItemNames"=w392:string[][])  [unwired: 2 in, 2 out]
        n148 = Variant To Data(error in=w396, type=string[] [], Variant=w397) -> (data=w391:string[], error out=w395:errorcluster)
        n149 = Build Array (concatenate)(w392, w391) -> (w389:string[][])
        n150 = property on="ErrorLog" class="MCListbox (strict)"("ItemNames"=w389) -> ()  [unwired: 2 in, 2 out]
        "ErrorIndicator" <- TRUE ("ErrorIndicator")
      }
      frame "Set Idling Display" {
        w398 = FALSE  # Visible
        w399 = TRUE  # Visible
        n151 = property on="Stop" class="Bool (strict)"("Visible"=w398) -> ()  [unwired: 2 in, 2 out]
        n152 = property on="Start" class="Bool (strict)"("Visible"=w399) -> ()  [unwired: 2 in, 2 out]
      }
      frame "Set Running Display" {
        w402 = TRUE  # Visible
        w403 = FALSE  # Visible
        n153 = property on="Stop" class="Bool (strict)"("Visible"=w402) -> ()  [unwired: 2 in, 2 out]
        n154 = property on="Start" class="Bool (strict)"("Visible"=w403) -> ()  [unwired: 2 in, 2 out]
      }
      frame "Clear Error History" {
        n155 = property on="ErrorLog" class="MCListbox (strict)"("ItemNames"=string[][] []) -> ()  [unwired: 2 in, 2 out]
        n156 = local write "ErrorIndicator"(FALSE ("ErrorIndicator")) -> ()
      }
      frame "Generate Error" {
      }
      frame "Set Tab" {
        n157 = Variant To Data(error in=w415, type=Tab."Eng Run Screen" ("Tab Control"), Variant=w417) -> (data=→"Tab Control":T14, error out=w414:errorcluster)
      }
    }
    n158 = Format Into String(format string="%s", initial string="3.UI Queue Handling\n", w362) -> (resulting string=w361:string)  [unwired: 1 in, 1 out]
    n159 = call "Error Control.vi"("Command"=ErrorCommand."Set Error", "error in (no error)"=w366, "Source"=w361) -> ()  [unwired: 5 in, 1 out]
    "UILoop" <- w363
  }
  n160 = local write "ErrorHandlingLoop"(w20) -> ()
  n161 = call "DisplayQ.vi"("command"=DisplayQCommand."Close", "error in (no error)"=w1) -> ("error out"=w3:errorcluster)  [unwired: 3 in, 3 out]
  n162 = call "StateQ.vi"("QueueCommand"=QueueCommand."Close", "error in (no error)"=w3) -> ("error out"=w5:errorcluster)  [unwired: 5 in, 1 out]
  n163 = local write "EventLoop"(w17) -> ()
  n164 = local write "UILoop"(w18) -> ()
  n165 = call "ErrorQ.vi"("command"=DisplayQCommand."Close", "error in (no error)"=w5) -> ("error out"=w6:errorcluster)  [unwired: 3 in, 3 out]
  n166 = call "SSDCExit.vi"("error in (no error)"=w6) -> ()  [unwired: 6 in, 1 out]
  n167 = local write "StateMachineLoop"(w19) -> ()
